vi "Navigation_Sensors.vi"(9 "car_theta":dbl, 10 "car_pos":dbl[](array[numeric]), 11 "output":dbl) -> (1 "output y(k)":dbl, 2 "min_dist":cdb, 3 "Theta_2":cdb)   [LabVIEW 2012]
uses:
  <vilib>/Simulation/Implementation/Shared/SIMSCR Execution Mode.ctl
  <vilib>/Simulation/Scripting/Companion Diagram/SimConfigNode/SimParams.ctl
  <vilib>/Simulation/Scripting/Companion Diagram/SimConfigNode/_simSolvers.ctl
  <vilib>/Simulation/Param Hierarchy/Typedefs/SIMPH Param Control Actions.ctl
  <vilib>/Simulation/Implementation/Shared/NILVSim_ParamChanged.vi
  <vilib>/Simulation/SignalArithmetic/Implementation/NILVSim Gain.llb/SIM Gain (scalar).vi
  <vilib>/Simulation/Utility/Implementation/NILVSim Memory.llb/NILVSim Memory (core).vi
  <vilib>/Simulation/ContinuousLinear/Implementation/NILVSim Transfer Function.llb/SIM Transfer Function Distributor (SISO).vi
  <vilib>/Simulation/ContinuousLinear/Implementation/NILVSim Transfer Function.llb/SIM Transfer Function Collector (SISO).vi
  <vilib>/Simulation/Implementation/Shared/NILVSim_Manager.vi
  <vilib>/Simulation/Implementation/Shared/NILVSim_FinalizeModel.vi
  <vilib>/Simulation/Implementation/Shared/SIM Unbundle Sim Info.vi
  <vilib>/Utility/error.llb/Clear Errors.vi
  <vilib>/Simulation/Implementation/Shared/NILVSim_GetModelError.vi
  <vilib>/Simulation/Implementation/Shared/SIM SimErrorHandler.vi
  <vilib>/Simulation/Implementation/Shared/SIM Bundle Sim Info.vi
  <vilib>/Simulation/Implementation/Shared/SIMSH Read Queue.vi
  <vilib>/Simulation/Implementation/Shared/NILVSim_Initialize.vi
  <vilib>/Simulation/Utility/Implementation/NILVSim Get Time and IsAcceptedStep.vi
  <vilib>/imath/engines/lvmath2/RunTimeEngine/ErrorHandling/NIMS_Finalize Error.vi
  <vilib>/imath/engines/lvmath2/RunTimeEngine/CommandStatement/NIMS_CommandStatement_MaskErr.vi
  <vilib>/imath/engines/lvmath2/RunTimeEngine/NodeEndStatement/NIMS_NodeEndStatement_Output.vi
  <instcachedir>/0/NIMS_NodeEndStatement_Output_53EC0D466D134D7ABD903AC30B43404B.lvgen/NIMS_NodeEndStatement_Output_53EC0D466D134D7ABD903AC30B43404B_010.vi
  <instcachedir>/0/NIMS_NodeEndStatement_Output_53EC0D466D134D7ABD903AC30B43404B.lvgen/NIMS_NodeEndStatement_Output_53EC0D466D134D7ABD903AC30B43404B_000.vi
  <instcachedir>/0/NIMS_NodeEndStatement_Output_53EC0D466D134D7ABD903AC30B43404B.lvgen/NIMS_NodeEndStatement_Output_53EC0D466D134D7ABD903AC30B43404B_005.vi
  <vilib>/imath/engines/lvmath2/RunTimeEngine/BuiltInFunctions/linramp/NIMS_linramp.vi
  <vilib>/imath/engines/lvmath2/RunTimeEngine/ArithmeticOperatorToken/NIMS_ArithmeticOperator_plus.vi
  <instcachedir>/0/NIMS_ArithmeticOperator_plus_8BD56D3B58F64DB5ABEB7224541A3CE7.lvgen/NIMS_ArithmeticOperator_plus_8BD56D3B58F64DB5ABEB7224541A3CE7_004.vi
  <vilib>/imath/engines/lvmath2/RunTimeEngine/ArithmeticOperatorToken/NIMS_ArithmeticOperator_times.vi
  <instcachedir>/0/NIMS_ArithmeticOperator_times_1C9874CB0A2E40D3A609F62CD8BBF4DC.lvgen/NIMS_ArithmeticOperator_times_1C9874CB0A2E40D3A609F62CD8BBF4DC_000.vi
  <vilib>/imath/engines/lvmath2/RunTimeEngine/ErrorHandling/NIMS_Create Error From Enums.vi
  <vilib>/imath/engines/lvmath2/RunTimeEngine/RangeToken/NIMS_Range_R2 - Integer.vi
  <instcachedir>/0/NIMS_Range_R2 - Integer_CD92A44154CA48D58B2F3E711AB114DB.lvgen/NIMS_Range_R2 - Integer_CD92A44154CA48D58B2F3E711AB114DB_000.vi
  <vilib>/imath/engines/lvmath2/RunTimeEngine/CommandStatement/MC_CommandStatement_break.vi
  <vilib>/imath/engines/lvmath2/RunTimeEngine/ReplaceToken/NIMS_Replace - Check Linear.vi
  <instcachedir>/0/NIMS_Replace - Check Linear_44ABB4D6A819426DBDF25CCE6827BF1D.lvgen/NIMS_Replace - Check Linear_44ABB4D6A819426DBDF25CCE6827BF1D_002.vi
  <vilib>/imath/engines/lvmath2/RunTimeEngine/VariableToken/Read/NIMS_Get Elements - RV(_) - Check.vi
  <instcachedir>/0/NIMS_Get Elements - RV(_) - Check_09E565EE58C54071A799578B82C9999A.lvgen/NIMS_Get Elements - RV(_) - Check_09E565EE58C54071A799578B82C9999A_000.vi
  <vilib>/imath/engines/lvmath2/RunTimeEngine/ReplaceToken/NIMS_Replace - Size Check _(_)=S.vi
  <instcachedir>/0/NIMS_Replace - Size Check _(_)=S_5AC8AA27B9694BB9828B57BCF666F597.lvgen/NIMS_Replace - Size Check _(_)=S_5AC8AA27B9694BB9828B57BCF666F597_001.vi
  <vilib>/imath/engines/lvmath2/RunTimeEngine/ReplaceToken/NIMS_Replace - V(S)=S.vi
  <instcachedir>/0/NIMS_Replace - V(S)=S_927EF1B21AA84780A9A306EC96B904EC.lvgen/NIMS_Replace - V(S)=S_927EF1B21AA84780A9A306EC96B904EC_001.vi
  <instcachedir>/0/NIMS_Get Elements - RV(_) - Check_09E565EE58C54071A799578B82C9999A.lvgen/NIMS_Get Elements - RV(_) - Check_09E565EE58C54071A799578B82C9999A_005.vi
  <vilib>/imathl/engines/lvmath/Functions/Error Handling/Create Error.vi
  <instcachedir>/0/NIMS_Replace - Check Linear_44ABB4D6A819426DBDF25CCE6827BF1D.lvgen/NIMS_Replace - Check Linear_44ABB4D6A819426DBDF25CCE6827BF1D_001.vi
  <instcachedir>/0/NIMS_Replace - Size Check _(_)=S_5AC8AA27B9694BB9828B57BCF666F597.lvgen/NIMS_Replace - Size Check _(_)=S_5AC8AA27B9694BB9828B57BCF666F597_000.vi
  <instcachedir>/0/NIMS_Replace - V(S)=S_927EF1B21AA84780A9A306EC96B904EC.lvgen/NIMS_Replace - V(S)=S_927EF1B21AA84780A9A306EC96B904EC_000.vi
  <vilib>/imath/engines/lvmath2/RunTimeEngine/BuiltInFunctions/abs/NIMS_abs(signed).vi
  <instcachedir>/0/NIMS_abs(signed)_C4FCB8E6058B49B797C7C8D53CA5F6EC.lvgen/NIMS_abs(signed)_C4FCB8E6058B49B797C7C8D53CA5F6EC_000.vi
  <vilib>/imath/engines/lvmath2/RunTimeEngine/ArithmeticOperatorToken/NIMS_ArithmeticOperator_power(S).vi
  <instcachedir>/0/NIMS_ArithmeticOperator_power(S)_5B050855CD444015B09DC7CA12D55B8A.lvgen/NIMS_ArithmeticOperator_power(S)_5B050855CD444015B09DC7CA12D55B8A_010.vi
  <vilib>/imath/engines/lvmath2/RunTimeEngine/BuiltInFunctions/asin/NIMS_asin(C).vi
  <instcachedir>/0/NIMS_asin(C)_F3E14D7F5FA648E9BF65D5738488DD5F.lvgen/NIMS_asin(C)_F3E14D7F5FA648E9BF65D5738488DD5F_001.vi
  <instcachedir>/0/NIMS_abs(signed)_C4FCB8E6058B49B797C7C8D53CA5F6EC.lvgen/NIMS_abs(signed)_C4FCB8E6058B49B797C7C8D53CA5F6EC_002.vi
  <vilib>/imath/engines/lvmath2/RunTimeEngine/BuiltInFunctions/min/2 inputs/NIMS_min(RG,RG)-no size check.vi
  <instcachedir>/0/NIMS_min(RG,RG)-no size check_7F67BAB91AFC452D9517D2EA1C8F5F88.lvgen/NIMS_min(RG,RG)-no size check_7F67BAB91AFC452D9517D2EA1C8F5F88_001.vi
  <vilib>/Simulation/Scripting/Companion Diagram/SimConfigNode/SimDog.xnode
  <vilib>/Simulation/Implementation/XNodeFramework/SimXNode/SimX.xnode
  <vilib>/Simulation/ContinuousLinear/Implementation/NILVSim Transfer Function.llb/SIM Transfer Function (SISO).vi
  <vilib>/Simulation/Implementation/Shared/NI_SIM_Implementation.lvlib
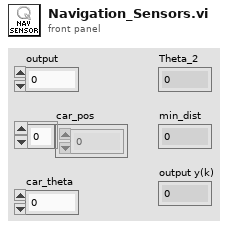
[diagram p1: front panel]
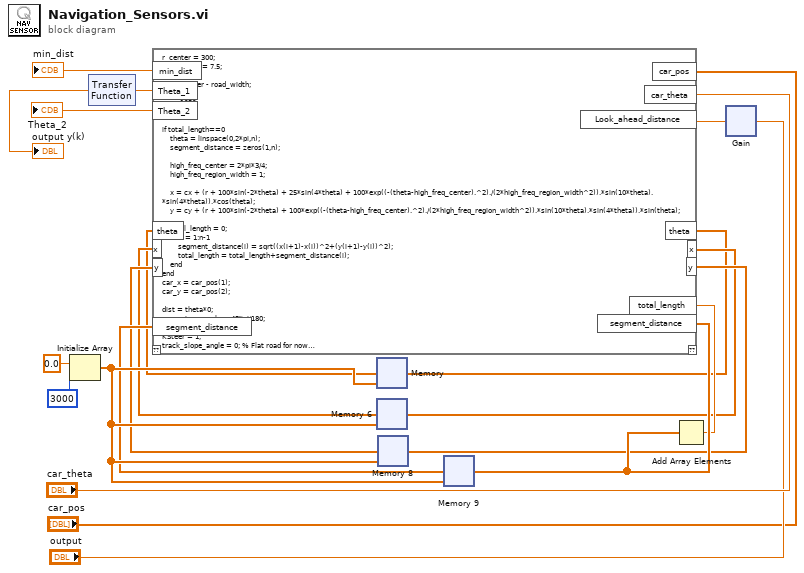
[diagram p0: block diagram]
diagram:
  n1 = Initialize Array(0.0 ("element"), 3000 ("dimension size")) -> (w14:dbl[])
  n2 = xnode ("Gain")("input"="output") -> ("output"=w2:dbl)  [unwired: 3 in]
  n3 = xnode ("Transfer Function")("input u(k)"=w3) -> ("output y(k)"=→"output y(k)":dbl)  [unwired: 3 in, 1 out]
  n4 = mathscript code="r_center = 300;\nroad_width = 7.5;\n\nr = r_center - road_width;\ncx = 900;\ncy = 1050;\nn = 3000;\n\nif total_length==0\n    theta = linspace(0,2*pi,n); \n    segment_distance = zeros(1,n);\n\n    high_freq_center = 2*pi*3/4;\n    high_freq_region_width = 1;\n\n    x = cx + (r + 100*sin(-2*theta) + 25*sin(4*theta) + 100*exp((-(theta-high_freq_center).^2)./(2*high_freq_region_width^2)).*sin(10*theta).*sin(4*theta)).*cos(theta);\n    y = cy + (r + 100*sin(-2*theta) + 100*exp((-(theta-high_freq_center).^2)./(2*high_freq_region_width^2)).*sin(10*theta).*sin(4*theta)).*sin(theta);\n    \n    total_length = 0;\n    for i = 1:n-1\n        segment_distance(i) = sqrt((x(i+1)-x(i))^2+(y(i+1)-y(i))^2);\n        total_length = total_length+segment_distance(i);\n    end\nend\ncar_x = car_pos(1);\ncar_y = car_pos(2);\n\ndist = theta*0;\nmax_steer_angle = 45*pi/180;\n\nKSteer = 1;\ntrack_slope_angle = 0; % Flat road for now \n       \n% minimum distance to path    \nmin_dist = inf;\nindex = 1;\n\nfor k = 1:(n-1)\n    dist(k) = (car_x-x(k))^2+(car_y-y(k))^2; % removed sqrt since it is not require for comparison.\n    \n    if (dist(k) < min_dist)\n        min_dist = dist(k);\n        index = k;\n    end\nend;\n\n% which is the second closest, the one in front or behind?\nindex_p1 = index + 1;\nif (index_p1 > (n-1))\n    index_p1 = 1;\nend\n\nindex_n1 = index - 1;\nif (index_n1 == 0)\n    index_n1 = (n-1);\nend\n\nif (dist(index_p1) < dist(index_n1))\n    index_alt = index_p1;\n    look_ahead_index = index_alt;\nelse \n    index_alt = index_n1;\n    look_ahead_index = index + 1;\n    \n    if (look_ahead_index > (n-1))\n        look_ahead_index = 1;\n    end    \nend\n\n% Calculate parameters of a line in the form of Ax + By + C1 = 0;\n\nA = y(index_alt) - y(index);\nB = x(index) - x(index_alt);\nC1 = y(index)*x(index_alt) - y(index_alt)*x(index);\n\nmin_dist = abs(A*car_x + B*car_y + C1)/sqrt(A^2 + B^2);\n\n% positive or negative error dictated by distance from center to intersection of\n% perpendicular line -Bx + Ay + C2 = 0\n\nC2 = B*car_x - A*car_y;\n\nif (A == 0)\n    \n    ideal_x = car_x;\n    ideal_y = -C1/B;\n    \nelseif (B == 0)\n    ideal_x = -C1/A;\n    ideal_y = car_y;\n    \nelse\n    ideal_x = (C2*B-C1*A)/(A^2 + B^2);\n    ideal_y = -A/B*ideal_x - C1/B;\nend\n\ncenter_to_car = (car_x - cx)^2 + (car_y - cy)^2;\ncenter_to_road = (ideal_x - cx)^2 + (ideal_y - cy)^2;\n\nif (center_to_car < center_to_road)\n    min_dist = -min_dist;\nend\n\n% Find point on road min distance ahead of current ideal car position on road (min_dist)\n\nindex_distance = sqrt( (x(look_ahead_index) - ideal_x)^2 + (y(look_ahead_index) - ideal_y)^2);\n\nwhile (index_distance < Look_ahead_distance)\n    look_ahead_index = look_ahead_index + 1;\n    if (look_ahead_index > (n-1))\n        look_ahead_index = 1;\n    end\n    \n    index_distance = index_distance + segment_distance(look_ahead_index);\n    \nend\n\nxahead = x(look_ahead_index);\nyahead = y(look_ahead_index);\n\n% Get the angle between looka ahead point and car direction vector \nVd_x = total_length*cos(car_theta);\nVd_y = total_length*sin(car_theta);\n\n% normalize \nMVd = (sqrt(Vd_x^2 + Vd_y^2));\nVd_x = Vd_x/MVd;\nVd_y = Vd_y/MVd;\n\nVe_x = xahead-car_x;\nVe_y = yahead-car_y;\nMVe = (sqrt(Ve_x^2 + Ve_y^2));\nVe_x = Ve_x/MVe;\nVe_y = Ve_y/MVe;\n\nCross_p = Vd_x*Ve_y-Ve_x*Vd_y;\n\nTheta_corr = -asin(Cross_p); \nTheta_1 = -KSteer*Theta_corr;\nTheta_1 = sign(Theta_1)*min(abs(Theta_1),max_steer_angle);\n\n% tangent vector at look ahead point\n% n_ahead is index at that point\n\nn_ahead = look_ahead_index;\n\nnext_x = 0;\nnext_y = 0;\nif(n_ahead<(n-1))\n    next_x = x(n_ahead+1);\n    next_y = y(n_ahead+1);\nend;\nif(n_ahead == (n-1))\n    next_x = x(1);\n    next_y = y(1);\nend;\n\nVt_x = x(n_ahead)-next_x;\nVt_y = y(n_ahead)-next_y;\nMVt = (sqrt(Vt_x^2 + Vt_y^2));\nVt_x = Vt_x/MVt;\nVt_y = Vt_y/MVt;\n\n% Get the angle betwen car direction and look ahead tangent \n\nCross_p = Vd_x*Vt_y-Vt_x*Vd_y;\nTheta_2 = -asin(Cross_p);"("car_pos"="car_pos", "car_theta"="car_theta", "Look_ahead_distance"=w2, "theta"=w7, "x"=w10, "y"=w11, "total_length"=w16, "segment_distance"=w17) -> ("theta"=w8:dbl[], "x"=w9:dbl[], "y"=w12:dbl[], "segment_distance"=w13:cdb[], "min_dist"=→"min_dist":cdb, "Theta_1"=w3:cdb, "Theta_2"=→"Theta_2":cdb)  [unwired: 1 in, 1 out]
  n5 = xnode ("Memory")("input"=w8, "initial value"=w14) -> ("output"=w7:dbl[])  [unwired: 4 in]
  n6 = xnode ("Memory 6")("input"=w9, "initial value"=w14) -> ("output"=w10:dbl[])  [unwired: 4 in]
  n7 = xnode ("Memory 8")("input"=w12, "initial value"=w14) -> ("output"=w11:dbl[])  [unwired: 4 in]
  n8 = xnode ("Memory 9")("input"=w13, "initial value"=w14) -> ("output"=w17:dbl[])  [unwired: 4 in]
  n9 = Add Array Elements(numeric array=w17) -> (sum=w16:dbl)
